vi "Write isOpen.vi"(8 "error in (no error)":errorcluster, 10 "isOpen":bool, 11 "Door in":refnum<class "Door.lvclass">) -> (0 "error out":errorcluster, 3 "Door out":refnum<class "Door.lvclass">)   [LabVIEW 2016, in "Door.lvclass"]
uses:
  Door.lvclass
  Door.lvclass/Door.ctl
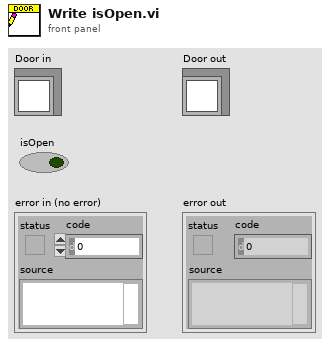
[diagram p1: front panel]
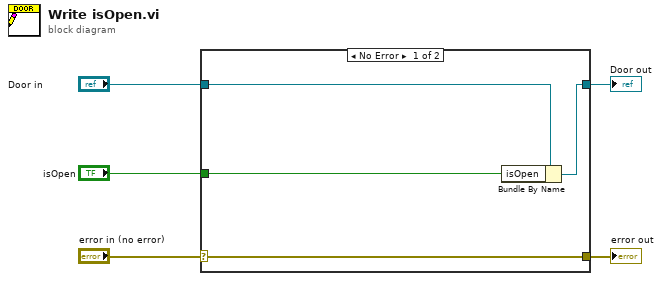
[diagram p0: block diagram]
diagram:
  n1 = case shown="No Error" "error in (no error)" {
    selector: "error in (no error)" -> [w9 w10]
    tunnel: [w9 w10] -> w4
    tunnel: [w7 w11] -> w2
    tunnel: "Door in" -> [w8 w11]
    tunnel: "isOpen" -> [w6 _]
    frame No Error {
      n2 = Bundle By Name(cluster=w8, "isOpen"=w6) -> (w7:refnum<class "Door.lvclass">)
    }
    frame Error {
    }
  }
  "error out" <- w4
  "Door out" <- w2
